vi "Move Frame Settings.vi"(8 "error in (no error)":errorcluster, 10 "Frames":T3(array[cluster]), 11 "Ref in":T1 format="%.0x") -> (0 "error out":errorcluster, 3 "Ref out":T1 format="%.0x")   [LabVIEW 2023, in "J1939 Addon System Explorer.lvlib"]
uses:
  J1939 Addon System Explorer.lvlib
  Addon Shared/Types/SPN Properties.ctl
  <vilib>/NI VeriStand/Custom Device API/Custom Device Item Ref.ctl
  <vilib>/NI VeriStand/Custom Device API/Custom Device Channel.ctl
  <vilib>/NI VeriStand/Custom Device API/Custom Device Channel Type.ctl
  Addon Shared/SubVIs/Constants.vi
  Addon Shared/J1939 Addon Shared.lvlib
  <vilib>/NI VeriStand/Custom Device API/Custom Device API.lvlib
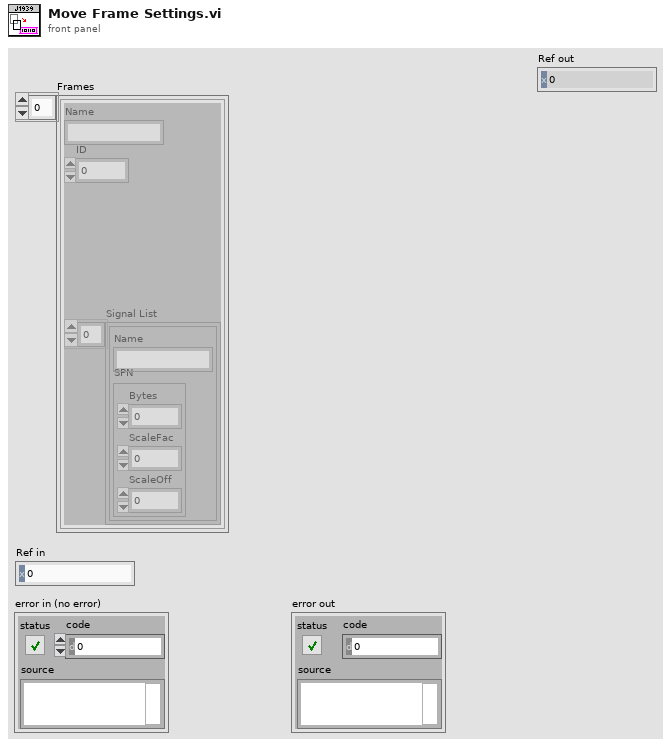
[diagram p1: front panel]
types:
  T1 = typedef "Custom Device API.lvlib/Custom Device Item Ref.ctl" = u64
  T2 = typedef "J1939 Addon Shared.lvlib/SPN Properties.ctl" = cluster{"Bytes":u32, "ScaleFac":dbl, "ScaleOff":dbl}
  T3 = cluster{"Name":string, "ID":u32, "Signal List":cluster{"Name":string, "SPN":T2}[]}[]
  T4 = typedef "Custom Device API.lvlib/Custom Device Item Info.ctl" = cluster{"Name":string, "Is Channel":bool, "GUID":string, "Is Waveform":bool}
  T5 = typedef "Custom Device API.lvlib/Custom Device Channel.ctl" = cluster{"Type":T6, "Units":string, "Default Value":dbl, "Faultable":bool, "Scalable":bool}
  T6 = typedef "Custom Device API.lvlib/Custom Device Channel Type.ctl" = enum16{"Input", "Output"}
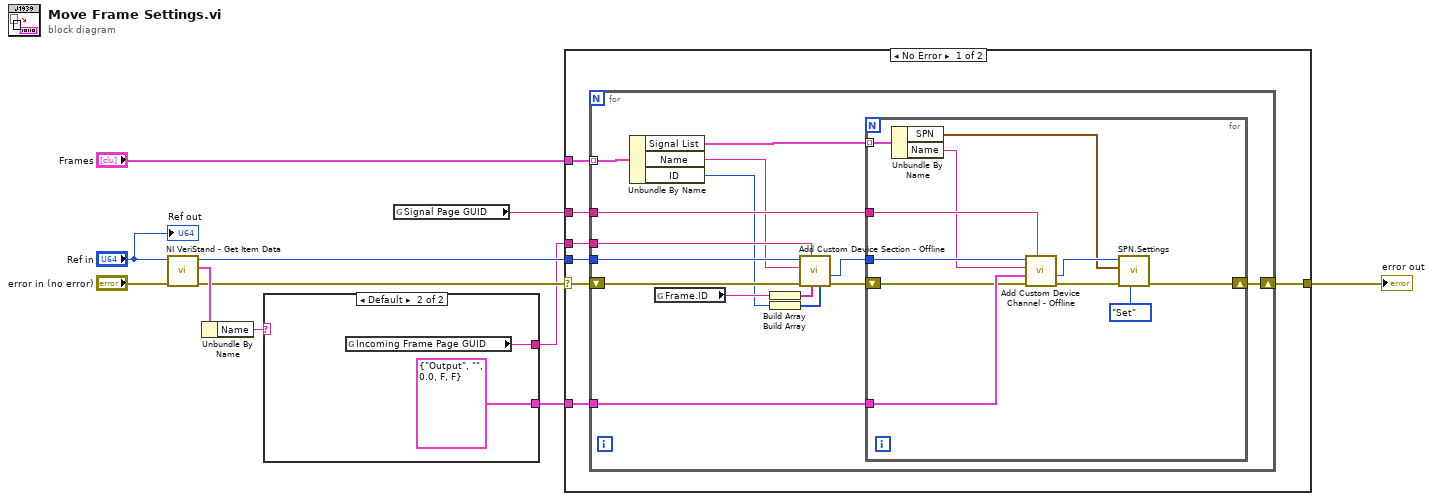
[diagram p0: block diagram]
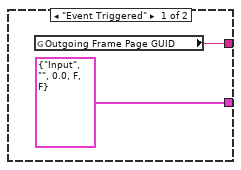
[diagram p2: hidden frame]
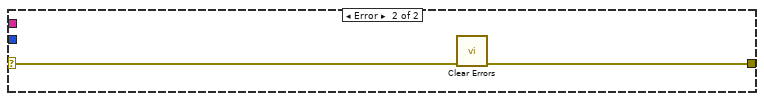
[diagram p3: hidden frame]
diagram:
  n1 = call <vilib>:"NI VeriStand - Get Item Data.vi"("error in (no error)"="error in (no error)", "Item Ref in"="Ref in") -> ("error out"=w3:errorcluster, "Item Info"=w6:T4, "Item Ref out"=w7:T1)  [unwired: 7 out]
  n2 = Unbundle By Name(w6) -> ("Name"=w5:string)
  n3 = case shown="Default" w5 {
    tunnel: [T5 {"Type"=enum."Input", "Units"="", "Default Value"=0.0, "Faultable"=FALSE, "Scalable"=FALSE} ("Channel") T5 {"Type"=enum."Output", "Units"="", "Default Value"=0.0, "Faultable"=FALSE, "Scalable"=FALSE} ("Channel")] -> w4
    tunnel: [w12 w14] -> w2
    frame "Event Triggered" {
      n4 = global read "Constants.vi" "Outgoing Frame Page GUID"() -> (w12:string)
    }
    frame Default {
      n5 = global read "Constants.vi" "Incoming Frame Page GUID"() -> (w14:string)
    }
  }
  n6 = global read "Constants.vi" "Signal Page GUID"() -> (w1:string)
  n7 = case shown="No Error" w3 {
    selector: w3 -> [w20 w50]
    tunnel: [w22 w49] -> w8
    tunnel: w7 -> [w21 _]
    tunnel: w1 -> [w19 _]
    tunnel: w2 -> [w18 _]
    tunnel: w4 -> [w17 _]
    tunnel: "Frames" -> [w16 _]
    frame No Error {
      n8 = for {
        shift-right: [w37] -> w22
        shift-left: w20 -> [w27]
        tunnel: w21 -> [w36]
        tunnel: w19 -> [w34]
        tunnel: w18 -> [w33]
        tunnel: w17 -> [w32]
        tunnel: w16 -> [w28] mode=indexing
        n9 = Unbundle By Name(w28) -> ("Signal List"=w29:cluster{"Name":string, "SPN":T2}[], "Name"=w25:string, "ID"=w26:u32)
        n10 = global read "Constants.vi" "Frame.ID"() -> (w35:string)
        n11 = Build Array(w35) -> (w30:string[])
        n12 = Build Array(w26) -> (w31:u32[])
        n13 = call "Add Custom Device Section - Offline.vi"("Property Values"=w31, "Property names"=w30, "GUID (Default Section)"=w33, "error in (no error)"=w27, "Section Name"=w25, "Parent Ref in"=w36) -> ("error out"=w24:errorcluster, "Section Ptr"=w23:T1)  [unwired: 2 in, 2 out]
        n14 = for {
          tunnel: w34 -> [w48]
          tunnel: w32 -> [w47]
          tunnel: w23 -> [w45]
          shift-right: [w41] -> w37
          shift-left: w24 -> [w46]
          tunnel: w29 -> [w44] mode=indexing
          n15 = Unbundle By Name(w44) -> ("SPN"=w39:T2, "Name"=w43:string)
          n16 = call "Add Custom Device Channel - Offline.vi"("GUID (Default Channel)"=w48, "error in (no error)"=w46, "Channel"=w47, "Channel Name"=w43, "Parent Ref in"=w45) -> ("error out"=w42:errorcluster, "Channel Ref"=w40:T1)  [unwired: 3 in, 2 out]
          n17 = call "SPN.Settings.vi"("Action"=enum8{"Get", "Set"}."Set", "error in (no error)"=w42, "SPN.Settings"=w39, "Item Ref in"=w40) -> ("error out"=w41:errorcluster)  [unwired: 5 in, 2 out]
        }
      }
    }
    frame Error {
      n18 = call <vilib>:"Clear Errors.vi"("error in (no error)"=w50) -> ("error out"=w49:errorcluster)  [unwired: 5 in, 1 out]
    }
  }
  "error out" <- w8
  "Ref out" <- "Ref in"
